vi "1 bit read.vi"(4 "Min time SCL low (uSec)":u32, 5 "Min Time SCL high (uSec)":u32) -> (3 "Data bit":bool)   [LabVIEW 2013]
uses:
  <vilib>/rvi/eio/common/nirviEmuTemplateMethod_errors.vi
  <vilib>/eio/EIOMethodNode/EIOMethodNode.xnode
  <vilib>/eio/EIONode/EIONode.xnode
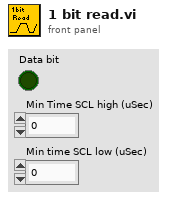
[diagram p1: front panel]
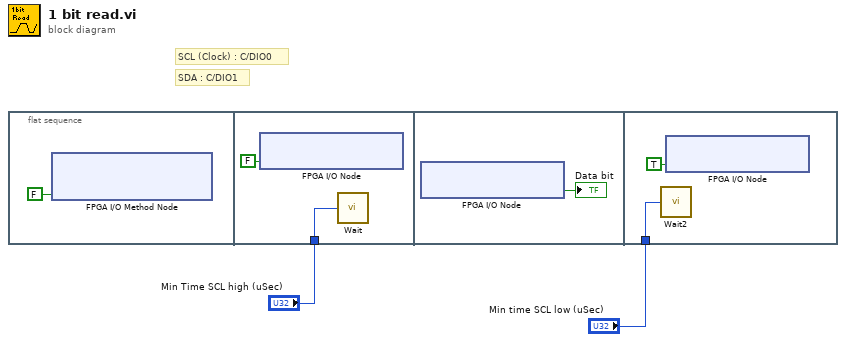
[diagram p0: block diagram]
diagram:
  # "SDA : C/DIO1"
  # "SCL (Clock) : C/DIO0"
  n1 = flat-sequence {
    tunnel: "Min Time SCL high (uSec)" -> [w4]
    tunnel: "Min time SCL low (uSec)" -> [w8]
    frame #0 {
      n2 = xnode "FPGA I/O Method Node"("Enable"=FALSE) -> ()  [unwired: 1 in, 1 out]
    }
    frame #1 {
      n3 = xnode "FPGA I/O Node"("ConnectorB/DIO12"=FALSE ("ConnectorC/DIO0")) -> ()  [unwired: 1 in, 1 out]
      n4 = call "Wait"("Count(uSec)"=w4) -> ()  [unwired: 1 out]
    }
    frame #2 {
      n5 = xnode "FPGA I/O Node"() -> ("ConnectorB/DIO13"=→"Data bit":bool)  [unwired: 1 in, 1 out]
    }
    frame #3 {
      n6 = call "Wait2"("Count(uSec)"=w8) -> ()  [unwired: 1 out]
      n7 = xnode "FPGA I/O Node"("ConnectorB/DIO12"=TRUE ("ConnectorC/DIO0")) -> ()  [unwired: 1 in, 1 out]
    }
  }
